vi "Unscale(Linear).vi"(9 "offset":dbl format="%#_13g", 10 "multiplier":dbl format="%#_13g", 11 "scaled value":dbl format="%#_13g") -> (3 "unscaled value":dbl)   [LabVIEW 2018, in "Scale.lvlib"]
uses:
  Scale.lvlib
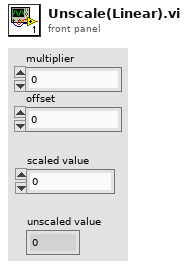
[diagram p1: front panel]
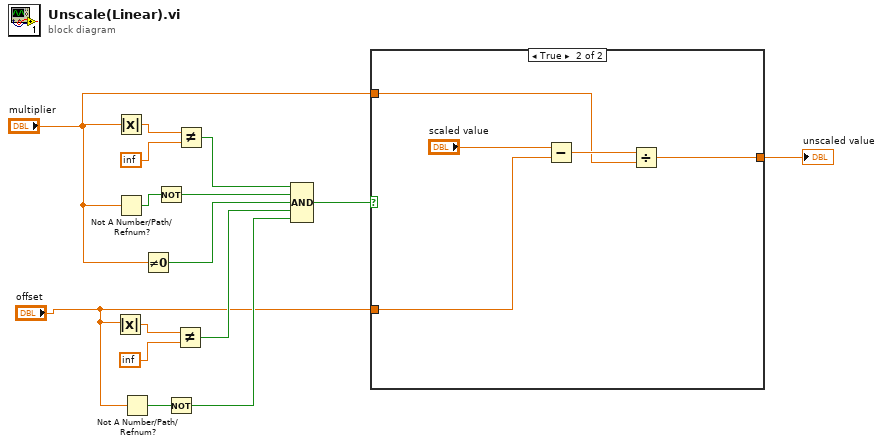
[diagram p0: block diagram]
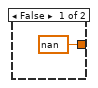
[diagram p2: hidden frame]
diagram:
  n1 = Absolute Value(x="offset") -> (abs(x)=w8:dbl)
  n2 = Absolute Value(x="multiplier") -> (abs(x)=w15:dbl)
  n3 = Not A Number/Path/Refnum?(number/path/refnum="multiplier") -> (NaN/Path/Refnum?=w12:bool)
  n4 = Not A Number/Path/Refnum?(number/path/refnum="offset") -> (NaN/Path/Refnum?=w7:bool)
  n5 = Not Equal To 0?(x="multiplier") -> (x != 0?=w10:bool)
  n6 = Not(x=w12) -> (.not. x?=w11:bool)
  n7 = Not(x=w7) -> (.not. x?=w5:bool)
  n8 = Not Equal?(x=w8, y=inf) -> (x != y?=w6:bool)
  n9 = Not Equal?(x=w15, y=inf) -> (x != y?=w13:bool)
  n10 = Compound Arithmetic op=AND(w13, w11, w10, w6, w5) -> (w2:bool)
  n11 = case shown="True" w2 {
    tunnel: "offset" -> [_ w19]
    tunnel: "multiplier" -> [_ w18]
    tunnel: [nan w17] -> w1
    frame False {
    }
    frame True {
      n12 = Subtract(x="scaled value", y=w19) -> (x-y=w20:dbl)
      n13 = Divide(x=w20, y=w18) -> (x/y=w17:dbl)
    }
  }
  "unscaled value" <- w1
